vi "Complex Outer Product PtByPt.vi"(0 "y":cdb format="%#.6g", 1 "sample length y":i32=10, 2 "x":cdb format="%#.6g", 3 "sample length x":i32=10, 4 "initialize":bool) -> (5 "Outer Product":cdb[][](array[numeric]), 6 "error":i32)   [LabVIEW 2020, in "NI_PtbyPt.lvlib"]
doc: "Computes the <B>Outer Product</B> of the complex values <B>y</B> and <B>x</B>."
uses:
  NI_PtbyPt.lvlib
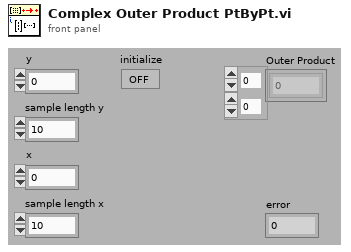
[diagram p1: front panel]
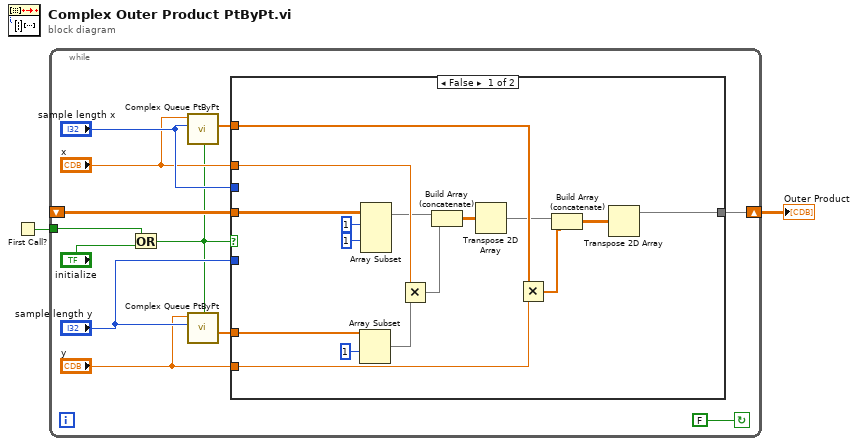
[diagram p0: block diagram]
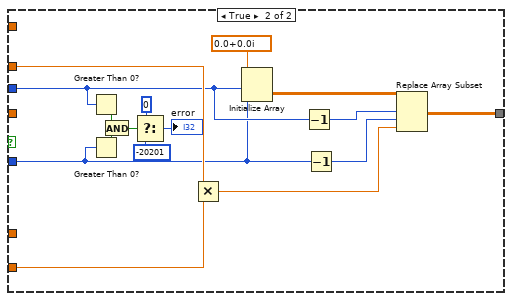
[diagram p2: hidden frame]
diagram:
  n1 = First Call?() -> (First Call?: T/F=w1:bool)
  n2 = while {
    tunnel: w1 -> [w5]
    shift-left: _ -> [w14]
    shift-right: [w13] -> w2
    stop <- FALSE continue-if-true
    n3 = Or(x=w5, y="initialize") -> (x .or. y?=w3:bool)
    n4 = call "Complex Queue PtByPt.vi"("initialize"=w3, "sample length"="sample length x", "input data point"="x") -> ("Current Queue"=w11:cdb[])  [unwired: 4 in, 4 out]
    n5 = call "Complex Queue PtByPt.vi"("initialize"=w3, "sample length"="sample length y", "input data point"="y") -> ("Previous Queue"=w12:cdb[])  [unwired: 4 in, 4 out]
    n6 = case shown="False" w3 {
      tunnel: w14 -> [w30 _]
      tunnel: [w29 w39] -> w13
      tunnel: w12 -> [w28 _]
      tunnel: "x" -> [w27 w46]
      tunnel: "y" -> [w26 w45]
      tunnel: w11 -> [w25 _]
      tunnel: "sample length y" -> [_ w37]
      tunnel: "sample length x" -> [_ w38]
      frame False {
        n7 = Array Subset(array=w28, index=1 ("Array Index")) -> (w20:cdb[])  [unwired: 1 in]
        n8 = Array Subset(array=w30, index (row)=1 ("Array Index"), index (col)=1 ("Array Index")) -> (w21:cdb[][])  [unwired: 2 in]
        n9 = Multiply(x=w27, y=w20) -> (x*y=w19:cdb[])
        n10 = Build Array (concatenate)(w21, w19) -> (w18:cdb[][])
        n11 = Transpose 2D Array(2D array=w18) -> (transposed array=w17:cdb[][])
        n12 = Multiply(x=w25, y=w26) -> (x*y=w16:cdb[])
        n13 = Build Array (concatenate)(w17, w16) -> (w15:cdb[][])
        n14 = Transpose 2D Array(2D array=w15) -> (transposed array=w29:cdb[][])
      }
      frame True {
        n15 = Greater Than 0?(x=w38) -> (x > 0?=w36:bool)
        n16 = Greater Than 0?(x=w37) -> (x > 0?=w35:bool)
        n17 = And(x=w36, y=w35) -> (x .and. y?=w34:bool)
        n18 = Select(t=0, s=w34, f=-20201) -> (s? t:f=→"error":i32)
        n19 = Multiply(x=w46, y=w45) -> (x*y=w42:cdb)
        n20 = Initialize Array(cdb 0.0+0.0i ("Element Data"), w38, w37) -> (w43:cdb[][])
        n21 = Decrement(x=w38) -> (x-1=w41:i32)
        n22 = Decrement(x=w37) -> (x-1=w40:i32)
        n23 = Replace Array Subset(array=w43, new element=w42, index (row)=w41, index (col)=w40) -> (w39:cdb[][])
      }
    }
  }
  "Outer Product" <- w2
